vi "Call by Reference Node.vi"() -> ()   [LabVIEW 2020]
panel:
  in  "Item":i32(listbox)
  in  "Exit":bool
  # "运行的模块"
  # "选择模块"
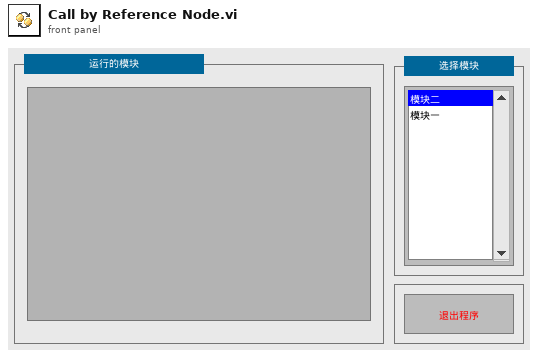
[diagram p1: front panel]
types:
  T1 = enum8{"Enabled", "Disabled", "Disabled and Grayed Out"}
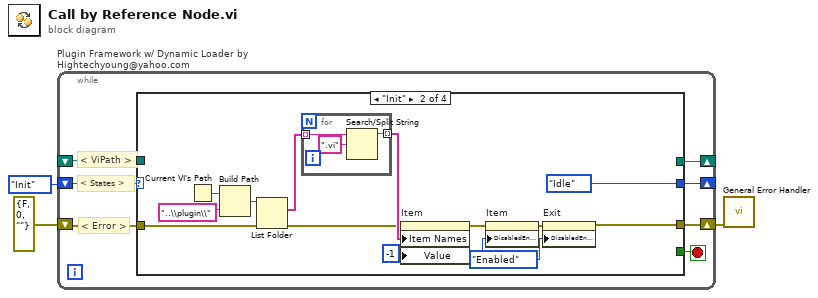
[diagram p0: block diagram]
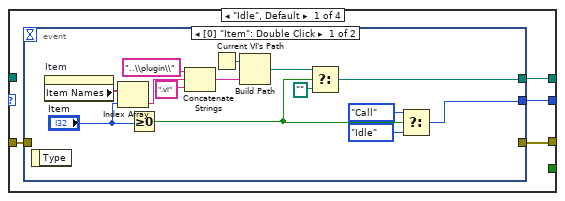
[diagram p2: hidden frame]
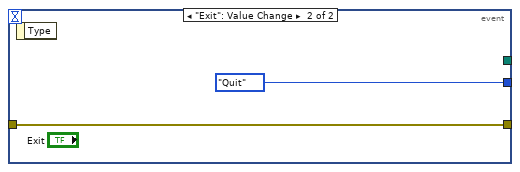
[diagram p3: hidden frame]
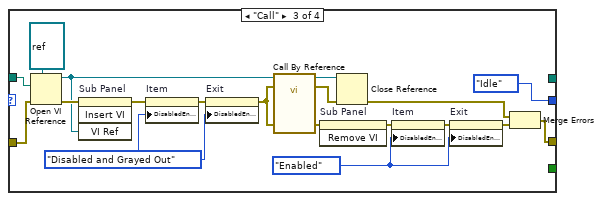
[diagram p4: hidden frame]
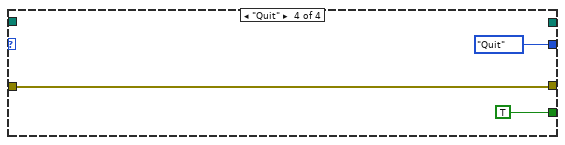
[diagram p5: hidden frame]
diagram:
  n1 = while "Plugin Framework w/ Dynamic Loader by Hightechyoung@yahoo.com" {
    shift-right: [w5] -> w3
    shift-left: errorcluster {"status"=FALSE, "code"=0, "source"=""} ("ErrorI") -> [w8]
    shift-right: [w9] -> _
    shift-left: enum16{"Idle", "Init", "Call", "Quit"}."Init" -> [w10]
    shift-right: [w6] -> _
    shift-left: _ -> [w4]
    stop <- w7 stop-if-true
    # "< Error >"
    # "< ViPath >"
    # "< States >"
    n2 = case shown="\"Init\"" w10 {
      tunnel: [w13 enum16{"Idle", "Init", "Call", "Quit"}."Idle" enum16{"Idle", "Init", "Call", "Quit"}."Idle" enum16{"Idle", "Init", "Call", "Quit"}."Quit"] -> w9
      tunnel: w8 -> [w14 w36 w59 w66]
      tunnel: [_ _ _ TRUE] -> w7
      tunnel: [w12 _ _ _] -> w6
      tunnel: [w11 w32 w55 w66] -> w5
      tunnel: w4 -> [_ _ w60 _]
      frame "Idle", Default {
        n3 = event shown="[0] \"Item\": Double Click" {
          selector: _ -> [_ _]
          dyn-events: _ -> [_ _]
          timeout: _ -> [_ _]
          tunnel: w14 -> [_ w29]
          tunnel: [w23 enum16{"Idle", "Init", "Call", "Quit"}."Quit"] -> w13
          tunnel: [w22 _] -> w12
          tunnel: [_ w29] -> w11
          event "Item": Double Click {
            n4 = event-data() -> ()  [unwired: 1 in, 1 out]
            n5 = property on="Item" class="LstBox (strict)"() -> ("Item Names"=w21:string[])  [unwired: 2 in, 2 out]
            n6 = Index Array(array=w21, index="Item") -> (element=w18:string)
            n7 = Greater Or Equal To 0?(x="Item") -> (x >= 0?=w26:bool)
            n8 = Concatenate Strings("..\\plugin\\" ("name or relative path"), w18, ".vi" ("string")) -> (w16:string)
            n9 = Current VI's Path() -> (path=w20:path)
            n10 = Build Path(base path=w20, name or relative path=w16) -> (appended path=w15:path)
            n11 = Select(t=w15, s=w26, f=path "") -> (s? t:f=w22:path)
            n12 = Select(t=enum16{"Idle", "Init", "Call", "Quit"}."Call", s=w26, f=enum16{"Idle", "Init", "Call", "Quit"}."Idle") -> (s? t:f=w23:enum16{"Idle", "Init", "Call", "Quit"})
          }
          event "Exit": Value Change {
            n13 = event-data() -> ()  [unwired: 1 in, 1 out]
          }
        }
      }
      frame "Init" {
        w31 = T1."Enabled" ("Disabled")
        n14 = Current VI's Path() -> (path=w40:path)
        n15 = Build Path(base path=w40, name or relative path="..\\plugin\\") -> (appended path=w39:path)
        n16 = List Folder(path=w39, error in=w36) -> (filenames=w37:string[], error out=w35:errorcluster)  [unwired: 2 in, 2 out]
        n17 = for {
          tunnel: w37 -> [w45] mode=indexing
          tunnel: [w44] -> w43 mode=indexing
          n18 = Search/Split String(string=w45, search string/char (-)=".vi" ("search string")) -> (substring before match=w44:string)  [unwired: 1 in, 2 out]
        }
        n19 = property on="Item" class="LstBox (strict)"(error in=w35, "Item Names"=w43, "Value"=-1 ("Item")) -> (error out=w33:errorcluster)  [unwired: 1 in, 1 out]
        n20 = property on="Item" class="LstBox (strict)"(error in=w33, "DisabledEnum"=w31) -> (error out=w34:errorcluster)  [unwired: 1 in, 1 out]
        n21 = property on="Exit" class="Bool"(error in=w34, "DisabledEnum"=w31) -> (error out=w32:errorcluster)  [unwired: 1 in, 1 out]
      }
      frame "Call" {
        w47 = T1."Disabled and Grayed Out" ("Disabled")
        w51 = T1."Enabled" ("Disabled")
        n22 = Open VI Reference(type specifier VI Refnum (for type only)=refnum<vi> refnum, vi path=w60, error in (no error)=w59) -> (vi reference=w56:refnum<vi>, error out=w63:errorcluster)  [unwired: 3 in]
        n23 = invoke on="Sub Panel" class="SubPanel" method="Insert VI"(error in=w63, "VI Ref"=w56) -> (error out=w54:errorcluster)  [unwired: 2 in, 3 out]
        n24 = property on="Item" class="LstBox (strict)"(error in=w54, "DisabledEnum"=w47) -> (error out=w49:errorcluster)  [unwired: 1 in, 1 out]
        n25 = property on="Exit" class="Bool"(error in=w49, "DisabledEnum"=w47) -> (error out=w48:errorcluster)  [unwired: 1 in, 1 out]
        n26 = call-by-ref "?"(reference=w56, error in=w48, "ErrorI"=w48) -> (reference out=w57:refnum<vi>, error out=w62:errorcluster, "ErrorO"=w64:errorcluster)  [unwired: 10 in]
        n27 = invoke on="Sub Panel" class="SubPanel" method="Remove VI"(error in=w64) -> (error out=w53:errorcluster)  [unwired: 2 in, 2 out]
        n28 = Close Reference(reference=w57, error in (no error)=w62) -> (error out=w65:errorcluster)
        n29 = property on="Item" class="LstBox (strict)"(error in=w53, "DisabledEnum"=w51) -> (error out=w52:errorcluster)  [unwired: 1 in, 1 out]
        n30 = property on="Exit" class="Bool"(error in=w52, "DisabledEnum"=w51) -> (error out=w50:errorcluster)  [unwired: 1 in, 1 out]
        n31 = Merge Errors(w65, w50) -> (w55:errorcluster)
      }
      frame "Quit" {
      }
    }
  }
  n32 = call <vilib>:"General Error Handler.vi"("error in (no error)"=w3) -> ()  [unwired: 10 in, 5 out]
